vi "Logging Merge Cache.vi"(1 "Update":T1, 2 "Cache":T1) -> (0 "Output":T1)   [LabVIEW 2012, in "femtoRoboLib.lvlib"]
uses:
  femtoRoboLib.lvlib
  Controls/Log Entry - Full Block.ctl
  Controls/Log Entry.ctl
  Controls/Log Value Type.ctl
  Controls/Log Value Cluster.ctl
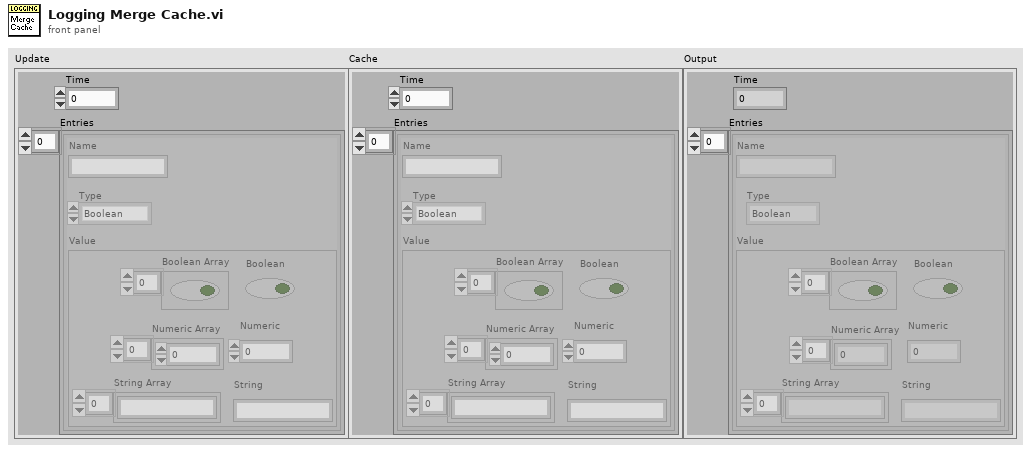
[diagram p1: front panel]
types:
  T1 = typedef "femtoRoboLib.lvlib/Log Entry - Full Block.ctl" = cluster{"Entries":T2[], "Time":u32}
  T2 = typedef "femtoRoboLib.lvlib/Log Entry.ctl" = cluster{"Name":string, "Type":T3, "Value":T4}
  T3 = typedef "femtoRoboLib.lvlib/Log Value Type.ctl" = enum16{"Boolean", "Numeric", "String", "Boolean Array", "Numeric Array", "String Array"}
  T4 = typedef "femtoRoboLib.lvlib/Log Value Cluster.ctl" = cluster{"Boolean Array":bool[], "Boolean":bool, "Numeric Array":dbl[], "Numeric":dbl, "String Array":string[], "String":string}
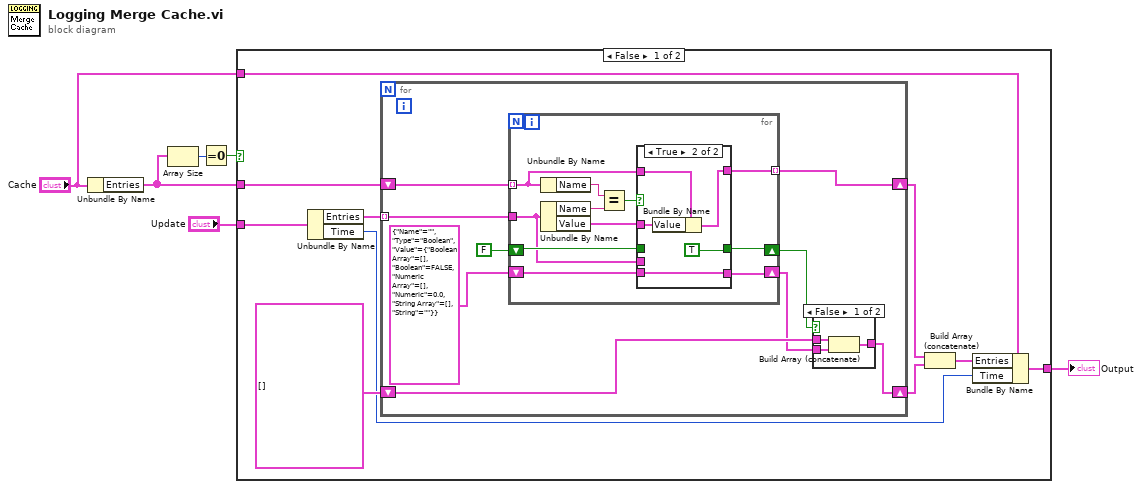
[diagram p0: block diagram]
diagram:
  n1 = Unbundle By Name("Cache") -> ("Entries"=w3:T2[])
  n2 = Array Size(array=w3) -> (size(s)=w2:i32)
  n3 = Equal To 0?(x=w2) -> (x = 0?=w1:bool)
  n4 = case shown="False" w1 {
    tunnel: "Update" -> [w16 w49]
    tunnel: [w11 w49] -> w5
    tunnel: "Cache" -> [w10 _]
    tunnel: w3 -> [w7 _]
    frame False {
      n5 = Unbundle By Name(w16) -> ("Entries"=w15:T2[], "Time"=w8:u32)
      n6 = for {
        tunnel: w15 -> [w24] mode=indexing
        shift-right: [w21] -> w12
        shift-left: T2[] [] -> [w18]
        shift-right: [w20] -> w13
        shift-left: w7 -> [w25]
        n7 = for {
          tunnel: w25 -> [w37] mode=indexing
          tunnel: w24 -> [w30]
          shift-right: [w31] -> w22
          shift-left: FALSE -> [w35]
          shift-right: [w34] -> w17
          shift-left: T2 {"Name"="", "Type"=enum."Boolean", "Value"={"Boolean Array"=[], "Boolean"=FALSE, "Numeric Array"=[], "Numeric"=0.0, "String Array"=[], "String"=""}} ("Log Variable") -> [w33]
          tunnel: [w32] -> w20 mode=indexing
          n8 = Unbundle By Name(w37) -> ("Name"=w39:string)
          n9 = Unbundle By Name(w30) -> ("Name"=w40:string, "Value"=w36:T4)
          n10 = Equal?(x=w39, y=w40) -> (x = y?=w38:bool)
          n11 = case shown="True" w38 {
            tunnel: w37 -> [w43 w48]
            tunnel: w36 -> [_ w47]
            tunnel: [w43 w46] -> w32
            tunnel: [w42 TRUE] -> w31
            tunnel: w35 -> [w42 _]
            tunnel: [w41 w44] -> w34
            tunnel: w33 -> [_ w44]
            tunnel: w30 -> [w41 _]
            frame False {
            }
            frame True {
              n12 = Bundle By Name(cluster=w48, "Value"=w47) -> (w46:T2)
            }
          }
        }
        n13 = case shown="False" w22 {
          tunnel: w18 -> [w28 w29]
          tunnel: [w27 w29] -> w21
          tunnel: w17 -> [w26 _]
          frame False {
            n14 = Build Array (concatenate)(w28, w26) -> (w27:T2[])
          }
          frame True {
          }
        }
      }
      n15 = Build Array (concatenate)(w13, w12) -> (w9:T2[])
      n16 = Bundle By Name(cluster=w10, "Entries"=w9, "Time"=w8) -> (w11:T1)
    }
    frame True {
    }
  }
  "Output" <- w5
